vi "Check OD Address.vi"(11 "Address":u16 format="%x") -> (3 "Support?":bool)   [LabVIEW 2021, in "CANOpen Addon System Explorer.lvlib"]
uses:
  CANOpen Addon System Explorer.lvlib
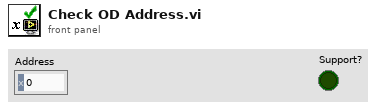
[diagram p1: front panel]
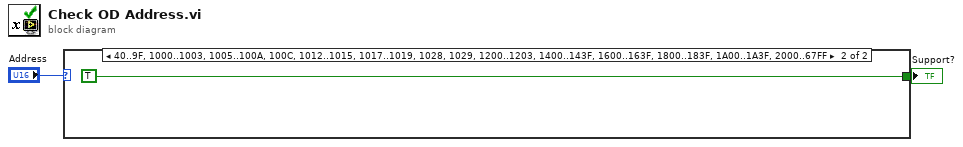
[diagram p0: block diagram]
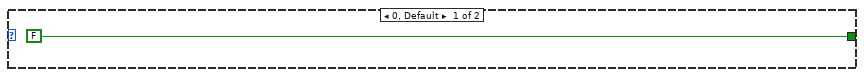
[diagram p2: hidden frame]
diagram:
  n1 = case shown="40..9F, 1000..1003, 1005..100A, 100C, 1012..1015, 1017..1019, 1028, 1029, 1200..1203, 1400..143F, 1600..163F, 1800..183F, 1A00..1A3F, 2000..67FF" "Address" {
    tunnel: [FALSE TRUE] -> w1
    frame 0, Default {
    }
    frame 64..159, 4096..4099, 4101..4106, 4108, 4114..4117, 4119..4121, 4136, 4137, 4608..4611, 5120..5183, 5632..5695, 6144..6207, 6656..6719, 8192..26623 {
    }
  }
  "Support?" <- w1
